vi "Get ByRef (DVR).vi"(8 "error in (no error)":errorcluster, 11 "Numeric in":refnum<class "Numeric Test Object.lvclass">) -> (0 "error out":errorcluster, 2 "Int":i32, 3 "Numeric out":refnum<class "Numeric Test Object.lvclass">)   [LabVIEW 2009, in "Numeric Test Object.lvclass"]
doc: "Gets the by-ref data held by the DVR."
uses:
  Numeric Test Object.lvclass
  Numeric Test Object.lvclass/Numeric Test Object.ctl
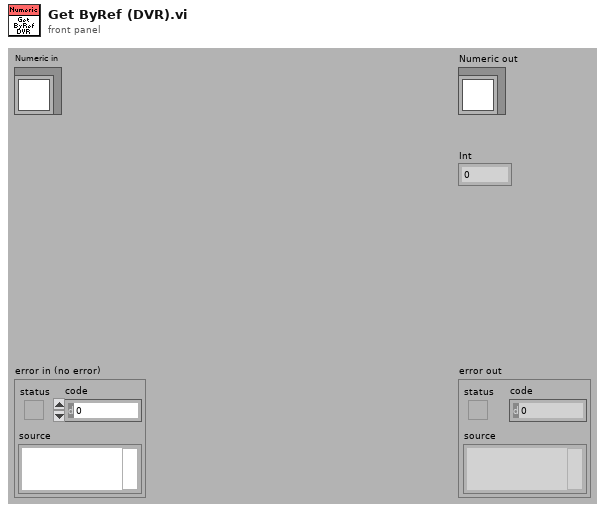
[diagram p1: front panel]
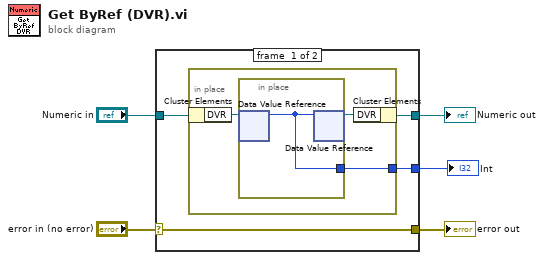
[diagram p0: block diagram]
diagram:
  n1 = case shown="No Error" "error in (no error)" {
    selector: "error in (no error)" -> [w9 w14]
    tunnel: [w9 w14] -> w4
    tunnel: [w7 w15] -> w2
    tunnel: "Numeric in" -> [w8 w15]
    tunnel: [w6 _] -> w1
    frame #0 {
      n2 = in-place {
        in-place-border: [w10] -> w6
        n3 = in-place-cluster #1(w8) -> ("DVR"=w12:refnum<data-value>)
        n4 = in-place {
          in-place-border: [w13] -> w10
          n5 = in-place-dvr #2(w12) -> (w13:i32)  [unwired: 1 out]
          n6 = in-place-dvr #2(w13) -> (w11:refnum<data-value>)  [unwired: 1 out]
        }
        n7 = in-place-cluster #1("DVR"=w11) -> (w7:refnum<class "Numeric Test Object.lvclass">)
      }
    }
    frame #1 {
    }
  }
  "error out" <- w4
  "Numeric out" <- w2
  "Int" <- w1
